vi "SegmentFile.vi"(8 "error in (no error)":errorcluster, 11 "Channel Manager in":refnum<class "Channel Manager.lvclass">) -> (0 "error out":errorcluster, 3 "Channel Manager out":refnum<class "Channel Manager.lvclass">)   [LabVIEW 2024, in "Embedded TDMS Logger Engine.lvlib" / "Channel Manager.lvclass"]
doc: "Checks whether the conditions for splitting up files is matched and if so, close the current file and start a new one."
uses:
  Channel Manager.lvclass
  Channel Manager.lvclass/Channel Manager.ctl
  Shared/File Classes/File/File.lvclass
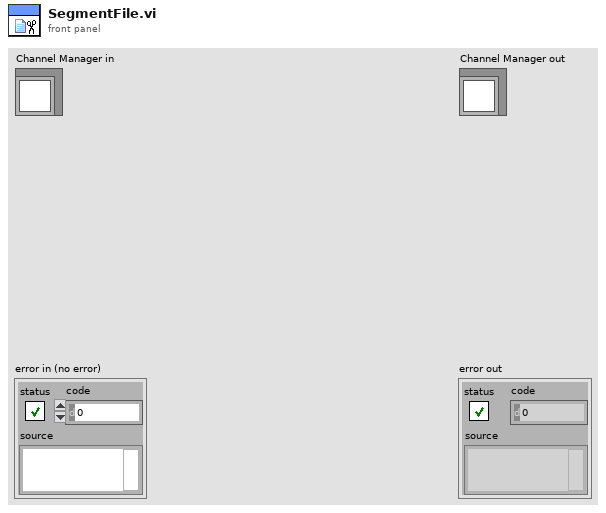
[diagram p1: front panel]
types:
  T1 = typedef "SegmentOptions.ctl" = enum16{"Time (s)", "Size (MB)"}
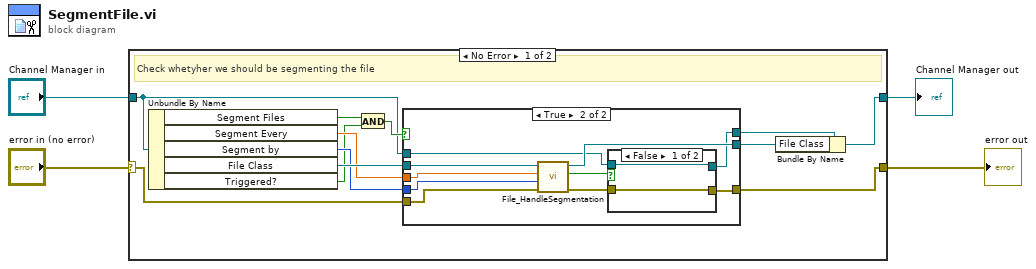
[diagram p0: block diagram]
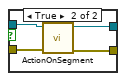
[diagram p3: hidden frame]
diagram:
  n1 = case shown="No Error" "error in (no error)" {
    selector: "error in (no error)" -> [w13 w37]
    tunnel: [w12 w37] -> w3
    tunnel: [w10 w36] -> w1
    tunnel: "Channel Manager in" -> [w6 w36]
    frame No Error {
      # "Check whetyher we should be segmenting the file"
      n2 = Unbundle By Name(w6) -> ("Segment Files"=w8:bool, "Segment Every"=w15:dbl, "Segment by"=w14:T1, "File Class"=w16:refnum<class "File.lvclass">, "Triggered?"=w7:bool)
      n3 = And(x=w8, y=w7) -> (x .and. y?=w9:bool)
      n4 = case shown="True" w9 {
        tunnel: w16 -> [w19 w29]
        tunnel: w15 -> [_ w28]
        tunnel: w14 -> [_ w27]
        tunnel: w13 -> [w18 w26]
        tunnel: [w18 w22] -> w12
        tunnel: [w19 w25] -> w11
        tunnel: w6 -> [w17 w20]
        tunnel: [w17 w21] -> w5
        frame False {
        }
        frame True {
          n5 = call-dynamic "File_HandleSegmentation.vi"("error in (no error)"=w26, "Segment by"=w27, "Segment Every"=w28, "File in"=w29) -> ("error out"=w24:errorcluster, "Segment?"=w23:bool, "File out"=w25:refnum<class "File.lvclass">)  [unwired: 5 in]
          n6 = case shown="False" w23 {
            tunnel: w24 -> [w30 w35]
            tunnel: [w30 w34] -> w22
            tunnel: [w31 w33] -> w21
            tunnel: w20 -> [w31 w32]
            frame False {
            }
            frame True {
              n7 = call-dynamic "ActionOnSegment.vi"("error in (no error)"=w35, "Channel Manager in"=w32) -> ("error out"=w34:errorcluster, "Channel Manager out"=w33:refnum<class "Channel Manager.lvclass">)  [unwired: 8 in]
            }
          }
        }
      }
      n8 = Bundle By Name(cluster=w5, "File Class"=w11) -> (w10:refnum<class "Channel Manager.lvclass">)
    }
    frame Error {
    }
  }
  "error out" <- w3
  "Channel Manager out" <- w1
